vi "FXP_MPCControlLaw_singleAxis_N22.vi"(7 "ControlParams_distEst":T3={"umax"=3.0, "Ns_obs/cntrl"=0, "ref_f_VEC"=[0.0, 0.0], "du_max"=0.0}, 8 "yd_est_x":fxp<+/-,32,5>, 11 "QP_params":T2={"maxIter"=0, "nuN"=24, "Ns_mpc"=0, "-beta"=-0.9987945556640625, "beta+1"=1.9987945556640625}) -> (0 "del u_x":fxp<+/-,64,15>, 2 "u_k (un saturated)":fxp<+/-,32,5>)   [LabVIEW 2017]
uses:
  typeDefs/FXPControlParams_distEst.ctl
  fgm_pipiline/quadProgParams_pipe.ctl
  typeDefs/x_vec_type.ctl
  <vilib>/Platform/TimedLoop/XDataNode/timing_clust.ctl
  <vilib>/Platform/TimedLoop/XDataNode/nitl_modes.ctl
  <vilib>/Platform/TimedLoop/XDataNode/wakeup.ctl
  typeDefs/x_vec_bram.ctl
  <vilib>/rvi/Emulation/niFpgaSctlEmulationGetInTimedLoop.vi
  <vilib>/rvi/Emulation/niFpgaEmulationReportErrorSimple.vi
  <vilib>/rvi/Emulation/niFpgaGetClockAttributes.vi
  <vilib>/rvi/Emulation/niFpgaCriticalErrorInLSC.vi
  <vilib>/rvi/DataTransferAndStorage/Container/Common/niFpgaContainerExecOnDevCompGetState.vi
  <vilib>/rvi/Emulation/niFpgaEmulationIsFPGAContextNoSignature.vi
  <vilib>/rvi/DataTransferAndStorage/Container/Common/niFpgaContainerGetUniqueNameForEmu.vi
  <vilib>/rvi/Emulation/niFpgaProcessEmulError.vi
  <vilib>/rvi/errors/nirviReportUnexpectedCaseInternalError (U32).vi
  <vilib>/rvi/Memory/Memory_Emulation/niFpgaMemoryEmulationCacheClearOnFirstRun.vi
  <vilib>/rvi/Memory/Memory_Emulation/nirvimemoryEmulationManagerCache_MakeExclusive.vi
  <vilib>/rvi/Memory/Memory_Emulation/niFpgaMemoryEmulationValidateCache.vi
  <vilib>/rvi/Memory/Memory_Emulation/nirvimemoryEmulationManagerCache_InsertValue.vi
  <vilib>/Utility/error.llb/Clear Errors.vi
  <vilib>/rvi/Memory/Memory_Emulation/nirvimemoryEmulationManagerCache_ReleaseExclusive.vi
  <vilib>/rvi/Memory/Memory_Emulation/nirvimemoryEmulationManagerCache_GetValue.vi
  <vilib>/rvi/Memory/Memory_Emulation/nirvimemoryEmulationManagerCache_SetValue.vi
  <vilib>/rvi/Emulation/niFpgaSctlEmulationResourceMgr.vi
  <vilib>/Platform/TimedLoop/XDataNode/XDataNode.xnode
  <vilib>/rvi/FXPMathLib/FxpAdd/XNode/nifxpmath_Add.xnode
  <vilib>/rvi/DataTransferAndStorage/Container/XNode/niFpgaContainer.xnode
  <vilib>/rvi/Memory/Memory_Emulation/niFpgaMemoryEmulationRefIn.vi
  <vilib>/Platform/TimedLoop/XDataNode/XDNodeRunTimeDep.lvlib
  <vilib>/rvi/FXPMathLib/sim/FxpSim.dll
panel:
  out "xerr":T1
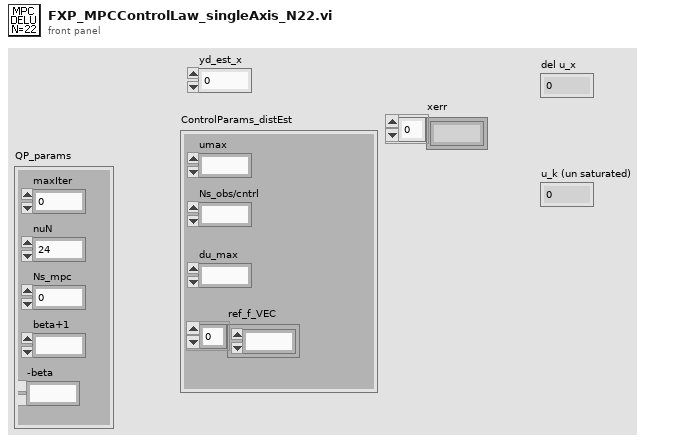
[diagram p1: front panel]
types:
  T1 = typedef "x_vec_type.ctl" = fxp<+/-,32,6>[]
  T2 = typedef "quadProgParams_pipe.ctl" = cluster{"maxIter":u16, "nuN":u16, "Ns_mpc":u16, "-beta":fxp<+/-,18,2>, "beta+1":fxp<+/-,18,2>}
  T3 = typedef "FXPControlParams_distEst.ctl" = cluster{"umax":fxp<+/-,18,5>, "Ns_obs/cntrl":u8, "ref_f_VEC":fxp<+/-,32,5>[], "du_max":fxp<+/-,18,5>}
  T4 = typedef "XDNodeRunTimeDep.lvlib/timing_clust.ctl" = cluster{"Expected End [f-1]":u64, "Actual End [f-1]":u64, "Finished Late? [f-1]":bool, "Expected End [i-1]":u64, "Actual End [i-1]":u64, "Finished Late? [i-1]":bool, "Expected Start [i]":u64, "Actual Start [i]":u64, "Expected Start [f]":u64, "Actual Start [f]":u64, "Source Name":string, "Structure Name":string, "Period":i64, "Deadline":i64, "Offset":i64, "Start":i64, "Priority":i32, "Timeout":i32, "Mode":T5, "Wakeup Reason":T6, "Error":errorcluster, "Source Type":string, "Secondary Source Type":string, "Global End Time":u64, "Global Start Time":u64, "Frame Duration":u64, "Iteration Duration":u64, "Assigned CPU":i32, "I/O Scan Engine Mode":u32}
  T5 = typedef "XDNodeRunTimeDep.lvlib/nitl_modes.ctl" = enum32{"No Change", "Process missed periods, maintain original phase", "Discard missed periods, maintain original phase", "Process missed periods, ignore original phase", "Discard missed periods, ignore original phase"}
  T6 = typedef "XDNodeRunTimeDep.lvlib/wakeup.ctl" = enum32{"Normal", "Aborted", "Asynchronous wakeup", "Timing source error", "Timed loop error", "Timeout"}
  T7 = typedef "x_vec_bram.ctl" = refnum<k21>
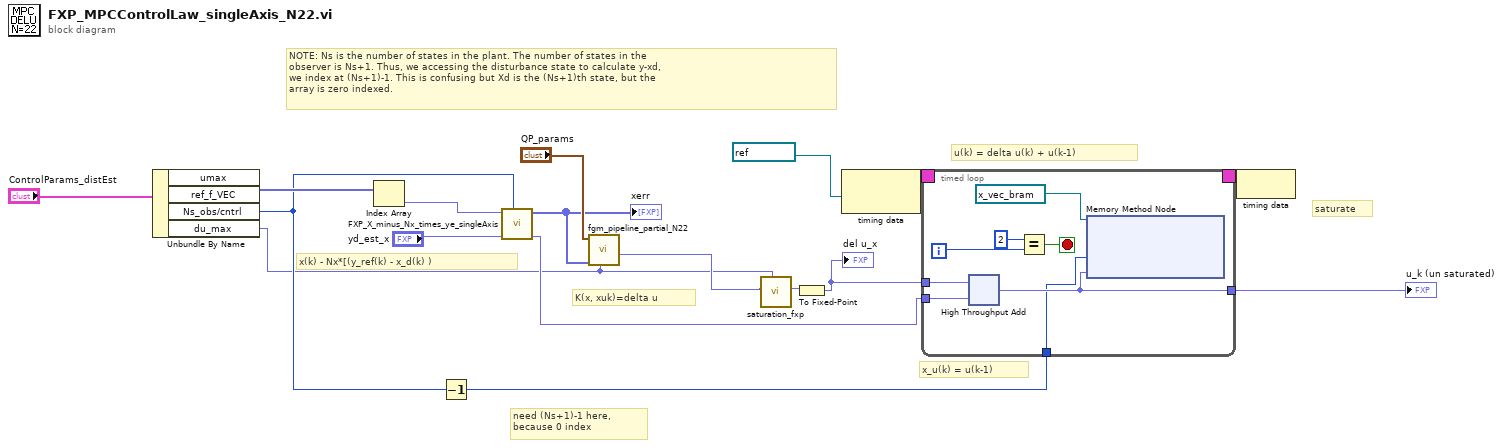
[diagram p0: block diagram]
diagram:
  # "saturate"
  # "need (Ns+1)-1 here,\nbecause 0 index"
  # "K(x, xuk)=delta u"
  # "u(k) = delta u(k) + u(k-1)"
  # "x_u(k) = u(k-1)"
  # "x(k) - Nx*[(y_ref(k) - x_d(k) )"
  # "NOTE: Ns is the number of states in the plant. The number of states in the \nobserver is Ns+1. Thus, we accessing the disturbance state to calculate y-xd, \nwe index at (Ns+1)-1. This is confusing but Xd is the (Ns+1)th state, but the \narray is zero indexed."
  n1 = Unbundle By Name("ControlParams_distEst") -> ("ref_f_VEC"=w14:fxp<+/-,32,5>[], "Ns_obs/cntrl"=w8:u8, "du_max"=w1:fxp<+/-,18,5>)  [unwired: 1 out]
  n2 = Index Array(array=w14) -> (element=w15:fxp<+/-,32,5>)  [unwired: 1 in]
  n3 = Decrement(x=w8) -> (x-1=w7:u8)
  n4 = call "FXP_X_minus_Nx_times_ye_singleAxis.vi"("NS"=w8, "yd_est_x"="yd_est_x", "ref(k)_x"=w15) -> ("xu_k"=w9:fxp<+/-,32,6>, "xerr"=w3:T1)  [unwired: 7 in]
  "xerr" <- w3
  n5 = call "fgm_pipeline_partial_N22.vi"("du_max"=w1, "x_vec"=w3, "QP_params"="QP_params") -> ("delta u(k)"=w2:fxp<+/-,32,3>)  [unwired: 6 in, 2 out]
  n6 = call "saturation_fxp.vi"("uMax"=w1, "signal_in"=w2) -> ("signal_out (saturated)"=w5:fxp<+/-,32,6>)  [unwired: 8 in, 1 out]
  n7 = To Fixed-Point(number=w5) -> (fixed-point=w13:fxp<+/-,32,6>)  [unwired: 1 in]
  "del u_x" <- w13
  n8 = node-c288(refnum<k21> "80MHz" ("Source Name")) -> (w12:T4)
  n9 = timed-loop {
    timing: w12 -> [_]
    timing-out: [_] -> w11
    tunnel: [w20] -> w6
    tunnel: w9 -> [w25]
    tunnel: w13 -> [w21]
    tunnel: w7 -> [w19]
    i -> [w23]
    stop <- w24 stop-if-true
    n10 = xnode ("High Throughput Add")("x"=w21, "y"=w25) -> ("x+y"=w20:fxp<+/-,32,5>)
    n11 = Equal?(x=2, y=w23) -> (x = y?=w24:bool)
    n12 = xnode ("Memory Method Node")("Address"=w19, "Data"=w20, "Memory In"=T7 "xk_1_2" ("Memory")) -> ()  [unwired: 1 out]
  }
  "u_k (un saturated)" <- w6
  n13 = node-c288(w11) -> ()
